vi "Read Indepenedent Label.vi"(9 "Page in":refnum<class "Page.lvclass">) -> (3 "Page out":refnum<class "Page.lvclass">, 4 "Indepenedent Label":bool)   [LabVIEW 2014, in "Page.lvclass"]
uses:
  Page.lvclass
  Page.lvclass/Page.ctl
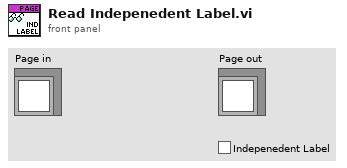
[diagram p1: front panel]
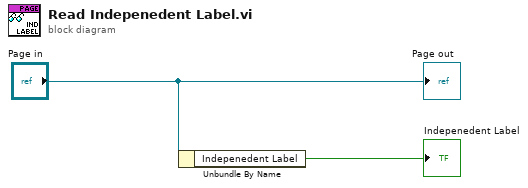
[diagram p0: block diagram]
diagram:
  n1 = Unbundle By Name("Page in") -> ("Indepenedent Label"=→"Indepenedent Label":bool)
  "Page out" <- "Page in"
